vi "Dialog Sample Container.vi"(8 "error in (no error)":errorcluster, 10 "Sample Clipboard Q":refnum<queue>, 11 "Container":T1) -> (0 "error out":errorcluster, 3 "Container out":T1)   [LabVIEW 2015, in "AMS UI.lvlib"]
doc: "Use this template to create a dialog box with event handling."
uses:
  AMS UI.lvlib
  Controls/Sample Container.ctl
  subs/Sample/Sample.lvclass
  subs/Sample/Sample.lvclass/Sample.ctl
  Controls/Ti Colors.ctl
  subs/Sample/Mixed Sample.vi
  <resource>/objmgr/ni.var.rc
panel:
  in  "Paste":bool
  in  "Copy":bool
  in  "Sample In":bool
  in  "OK Button":bool
  out "Color Box":u32(colorbox)
  in  "Clear":bool
  in  "Comment":string
  in  "Ti Cathode":i8 min=-1 max=39 step=1
  in  "Sample Name":string
  in  "Cancel":bool
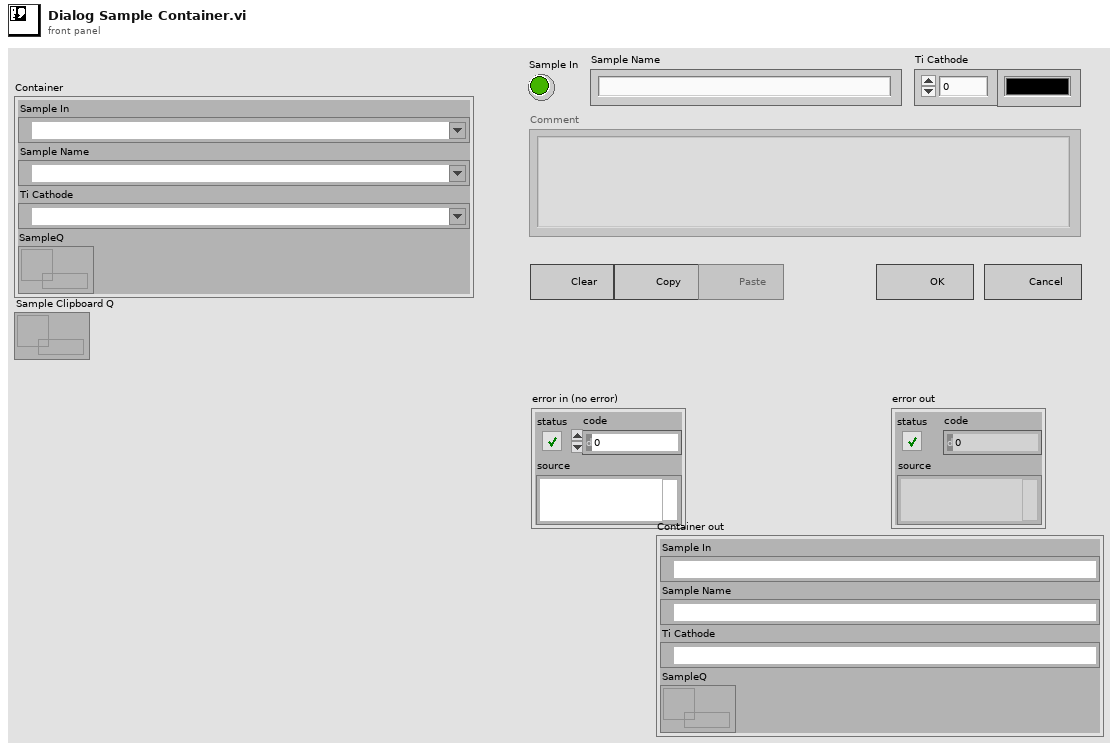
[diagram p1: front panel]
types:
  T1 = typedef "Sample Container.ctl" = cluster{"Sample In":refnum<k21>, "Sample Name":refnum<k21>, "Ti Cathode":refnum<k21>, "SampleQ":refnum<queue>}
  T2 = enum8{"Enabled", "Disabled", "Disabled and Grayed Out"}
  T3 = typedef "Ti Colors.ctl" = u32[]
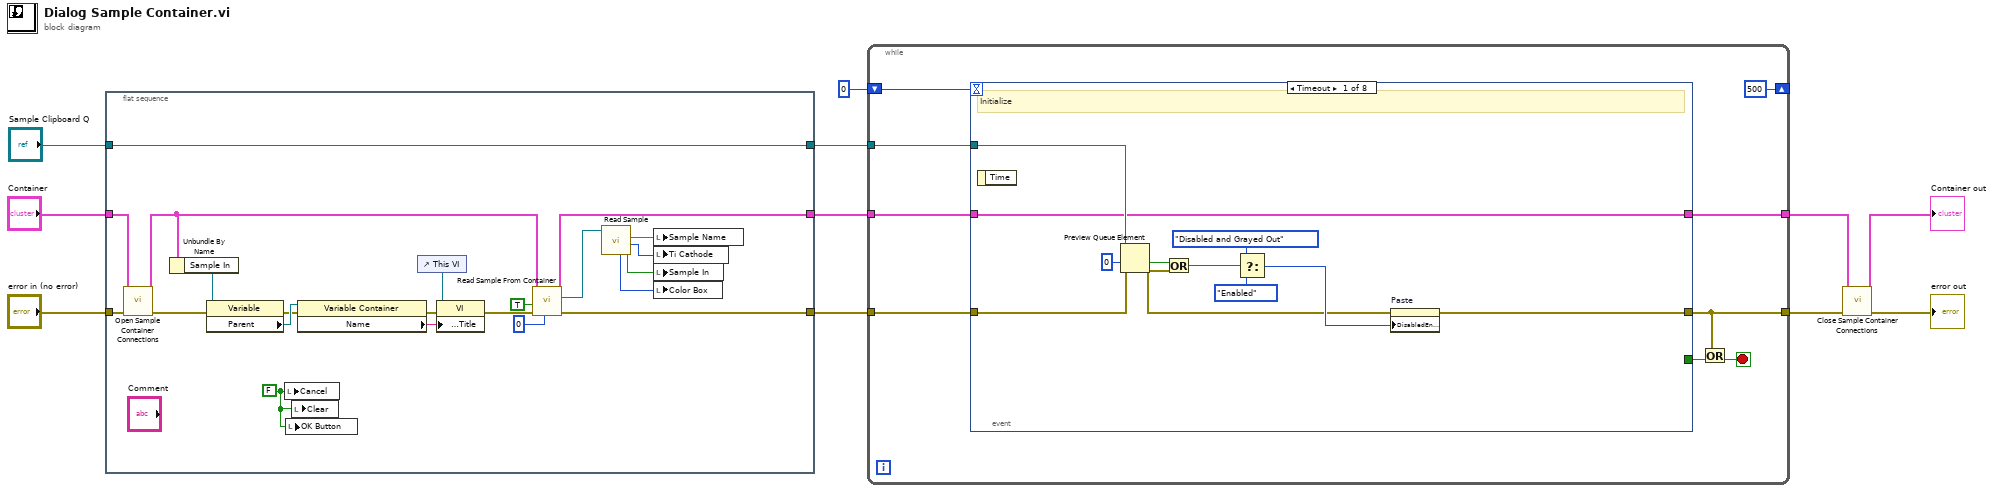
[diagram p0: block diagram]
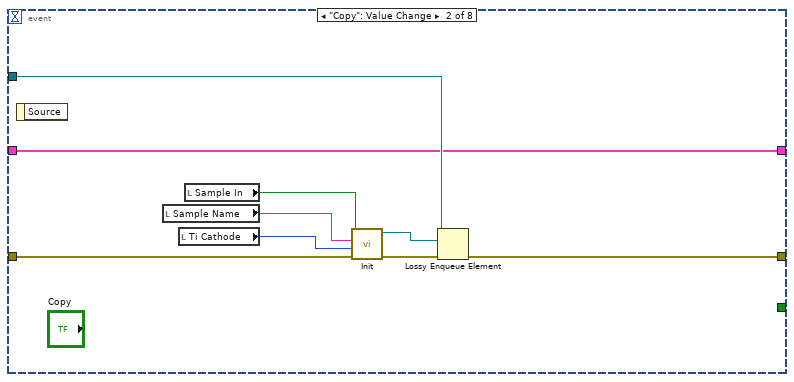
[diagram p2: hidden frame]
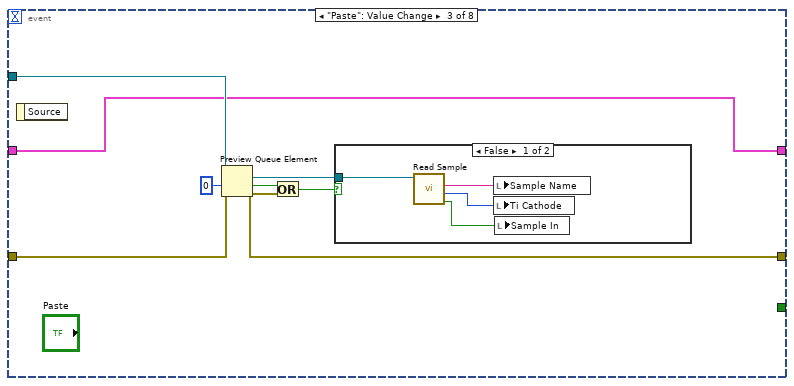
[diagram p3: hidden frame]
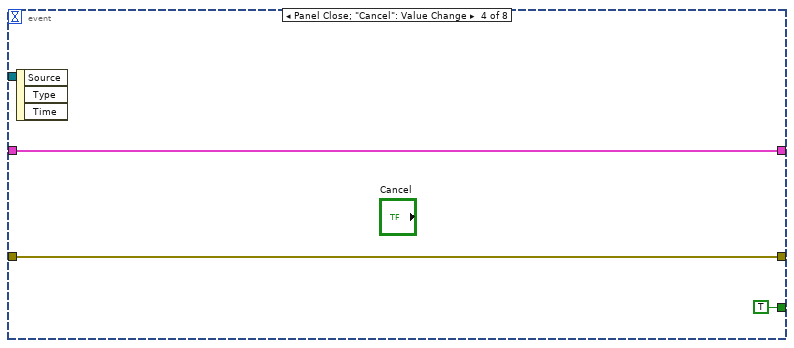
[diagram p5: hidden frame]
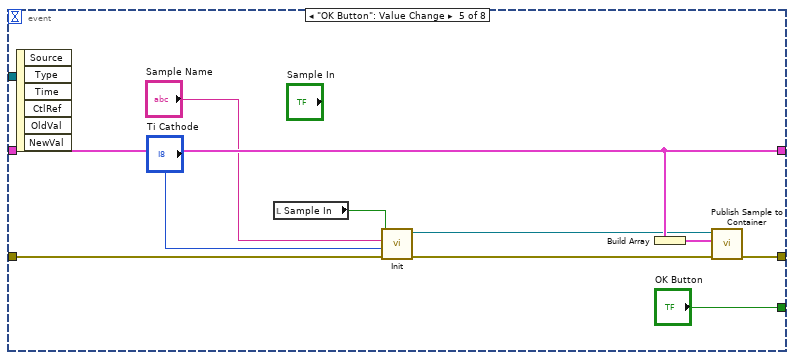
[diagram p6: hidden frame]
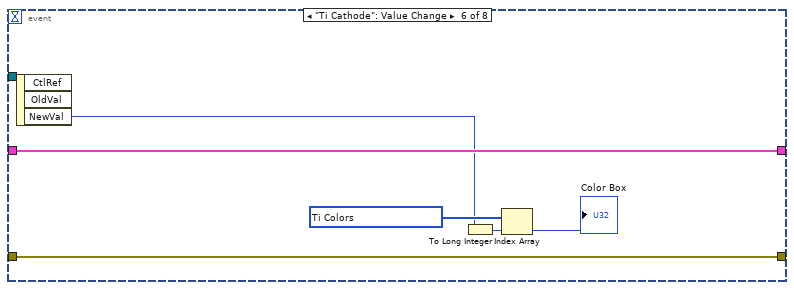
[diagram p7: hidden frame]
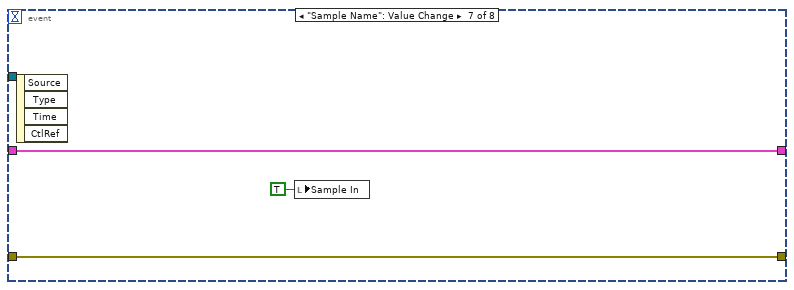
[diagram p8: hidden frame]
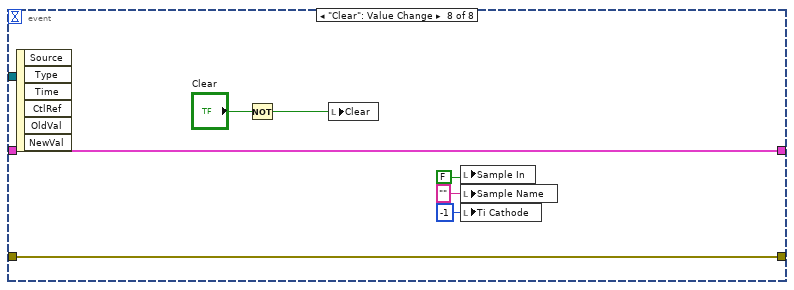
[diagram p9: hidden frame]
diagram:
  n1 = flat-sequence {
    tunnel: "error in (no error)" -> [w33]
    tunnel: [w15] -> w9
    tunnel: "Container" -> [w32]
    tunnel: [w13] -> w7
    tunnel: "Sample Clipboard Q" -> [w12]
    tunnel: [w12] -> w1
    frame #0 {
      w29 = FALSE ("Cancel")
      n2 = call "Open Sample Container Connections.vi"("error in (no error)"=w33, "Container in"=w32) -> ("error out"=w16:errorcluster, "Container out"=w14:T1)  [unwired: 8 in]
      n3 = Unbundle By Name(w14) -> ("Sample In"=w19:refnum<k21>)
      n4 = property class="Variable"(reference=w19, error in=w16) -> (error out=w20:errorcluster, "Parent"=w21:refnum<k21>)  [unwired: 1 out]
      n5 = local write "Cancel"(w29) -> ()
      n6 = local write "OK Button"(w29) -> ()
      n7 = local write "Clear"(w29) -> ()
      n8 = property class="Variable Container"(reference=w21, error in=w20) -> (error out=w22:errorcluster, "Name"=w24:string)  [unwired: 1 out]
      n9 = control-ref of="This VI"() -> (w23:refnum<vi>)
      n10 = property class="VI"(reference=w23, error in=w22, "Front Panel.Title"=w24) -> (error out=w25:errorcluster)  [unwired: 1 out]
      n11 = call "Read Sample From Container.vi"("Queue timeout in ms (-1)"=0, "error in (no error)"=w25, "Read from SHV (F)"=TRUE, "Container"=w14) -> ("error out"=w15:errorcluster, "Sample out"=w17:refnum<class "Sample.lvclass">, "Container"=w13:T1)  [unwired: 3 in, 2 out]
      n12 = call "Read Sample.vi"("Sample in"=w17) -> ("Sample In"=w31:bool, "Ti Cathode"=w27:i8, "Name"=w26:string, "Color"=w28:u32)  [unwired: 6 in, 1 out]
      n13 = local write "Sample Name"(w26) -> ()
      n14 = local write "Ti Cathode"(w27) -> ()
      n15 = local write "Sample In"(w31) -> ()
      n16 = local write "Color Box"(w28) -> ()
    }
  }
  n17 = while {
    shift-right: [500] -> _
    shift-left: 0 -> [w42]
    tunnel: w7 -> [w40]
    tunnel: w9 -> [w39]
    tunnel: [w36] -> w6
    tunnel: [w35] -> w4
    tunnel: w1 -> [w34]
    stop <- w37 stop-if-true
    n18 = event shown="[0] Timeout" {
      selector: _ -> [_ _ _ _ _ _ _ _]
      dyn-events: _ -> [_ _ _ _ _ _ _ _]
      timeout: w42 -> [_ _ _ _ _ _ _ _]
      tunnel: w40 -> [w49 w56 w68 w76 w85 w92 w95 w100]
      tunnel: w39 -> [w50 w62 w65 w75 w83 w93 w94 w101]
      tunnel: [w44 w54 w64 w75 w86 w93 w94 w101] -> w36
      tunnel: [_ _ _ TRUE "OK Button" _ _ _] -> w38
      tunnel: [w49 w56 w68 w76 w85 w92 w95 w100] -> w35
      tunnel: w34 -> [w53 w58 w70 _ _ _ _ _]
      event Timeout {
        # "Initialize"
        n19 = event-data() -> ()  [unwired: 1 in, 1 out]
        n20 = Preview Queue Element(queue=w53, timeout in ms (-1)=0, error in (no error)=w50) -> (timed out?=w51:bool, error out=w43:errorcluster)  [unwired: 2 out]
        n21 = Or(x=w51, y=w43) -> (x .or. y?=w48:bool)
        n22 = Select(t=T2."Disabled and Grayed Out", s=w48, f=T2."Enabled" ("Disabled")) -> (s? t:f=w45:T2)
        n23 = property on="Paste" class="Bool"(error in=w43, "DisabledEnum"=w45) -> (error out=w44:errorcluster)  [unwired: 1 in, 1 out]
      }
      event "Copy": Value Change {
        n24 = event-data() -> ()  [unwired: 1 in, 1 out]
        n25 = local read "Sample Name"() -> (w60:string)
        n26 = local read "Ti Cathode"() -> (w59:i8)
        n27 = local read "Sample In"() -> (w61:bool)
        n28 = call "Init.vi"("error in (no error)"=w62, "Ti Cathode"=w59, "Name"=w60, "Sample in"=w61) -> ("error out"=w55:errorcluster, "Sample out"=w57:refnum<class "Sample.lvclass">)  [unwired: 6 in]
        n29 = Lossy Enqueue Element(queue=w58, element=w57, error in (no error)=w55) -> (error out=w54:errorcluster)  [unwired: 3 out]
      }
      event "Paste": Value Change {
        n30 = event-data() -> ()  [unwired: 1 in, 1 out]
        n31 = Preview Queue Element(queue=w70, timeout in ms (-1)=0, error in (no error)=w65) -> (element=w66:refnum<class "Sample.lvclass">, timed out?=w69:bool, error out=w64:errorcluster)  [unwired: 1 out]
        n32 = Or(x=w69, y=w64) -> (x .or. y?=w67:bool)
        n33 = case shown="False" w67 {
          tunnel: w66 -> [w74 _]
          frame False {
            n34 = call "Read Sample.vi"("Sample in"=w74) -> ("Sample In"=w73:bool, "Ti Cathode"=w71:i8, "Name"=w72:string)  [unwired: 6 in, 2 out]
            n35 = local write "Sample Name"(w72) -> ()
            n36 = local write "Ti Cathode"(w71) -> ()
            n37 = local write "Sample In"(w73) -> ()
          }
          frame True {
          }
        }
      }
      event Panel Close; "Cancel": Value Change {
        n38 = event-data() -> ()  [unwired: 1 in, 3 out]
      }
      event "OK Button": Value Change {
        n39 = event-data() -> ()  [unwired: 1 in, 6 out]
        n40 = local read "Sample In"() -> (w78:bool)
        n41 = call "Init.vi"("error in (no error)"=w83, "Ti Cathode"="Ti Cathode", "Name"="Sample Name", "Sample in"=w78) -> ("error out"=w81:errorcluster, "Sample out"=w80:refnum<class "Sample.lvclass">)  [unwired: 6 in]
        n42 = Build Array(w85) -> (w84:T1[])
        n43 = call "Publish Sample to Container.vi"("error in (no error)"=w81, "Containers"=w84, "Sample in"=w80) -> ("error out"=w86:errorcluster)  [unwired: 7 in, 1 out]
      }
      event "Ti Cathode": Value Change {
        n44 = event-data() -> ("NewVal"=w89:i8)  [unwired: 1 in, 2 out]
        n45 = To Long Integer(number=w89) -> (32bit integer=w90:i32)
        n46 = Index Array(array=T3 [418898, 837796, 1256694, 1675592, 2094490, 2513388, 2932286, 3351184, 3770082, 4188980, 4607878, 5026776, 5445674, 5864572, 6283470, 6702368, 7121266, 7540164, 7959062, 8377960, 8796858, 9215756, 9634654, 10053552, 10472450, 10891348, 11310246, 11729144, 12148042, 12566940, 12985838, 13404736, 13823634, 14242532, 14661430, 15080328, 15499226, 15918124, 16337022, 16755920] ("output array 2"), index=w90) -> (element=→"Color Box":u32)
      }
      event "Sample Name": Value Change {
        n47 = event-data() -> ()  [unwired: 1 in, 4 out]
        n48 = local write "Sample In"(TRUE ("Sample In")) -> ()
      }
      event "Clear": Value Change {
        n49 = event-data() -> ()  [unwired: 1 in, 6 out]
        n50 = Not(x="Clear") -> (.not. x?=w97:bool)
        n51 = local write "Clear"(w97) -> ()
        n52 = local write "Sample In"(FALSE ("Sample In")) -> ()
        n53 = local write "Sample Name"("" ("Sample Name")) -> ()
        n54 = local write "Ti Cathode"(i8 -1 ("Ti Cathode")) -> ()
      }
    }
    n55 = Or(x=w36, y=w38) -> (x .or. y?=w37:bool)
  }
  n56 = call "Close Sample Container Connections.vi"("error in (no error)"=w6, "Container in"=w4) -> ("error out"=→"error out":errorcluster, "Container out"=→"Container out":T1)  [unwired: 8 in]
